vi "AcqLoop.vi"(8 "error in (no error)":errorcluster, 11 "Device in":refnum<class "Device.lvclass">) -> (0 "error out":errorcluster, 3 "Device out":refnum<class "Device.lvclass">)   [LabVIEW 2020, in "Device.lvlib" / "Device.lvclass"]
uses:
  Device.lvclass
  C:/Program Files/National Instruments/LabVIEW 2020/vi.lib/ActorFramework/Actor/Actor.lvclass
  DeviceStatus.ctl
  Device.lvclass/Device.ctl
  <vilib>/ActorFramework/Actor/Actor.lvclass/Actor.ctl
  <vilib>/ActorFramework/Message Enqueuer/Message Enqueuer.lvclass/Message Enqueuer.ctl
  <vilib>/ActorFramework/Message Enqueuer/Init from Existing Queue.vi
  <vilib>/ActorFramework/Message Enqueuer/Enqueue.vi
  Device Messages/AcqLoop Msg/AcqLoop Msg.lvclass
  C:/Program Files/National Instruments/LabVIEW 2020/vi.lib/ActorFramework/Message/Message.lvclass
  <vilib>/ActorFramework/Message Priority Queue/Priority Enqueue.vi
  <vilib>/ActorFramework/Message Enqueuer/Message Enqueuer.lvclass
  <vilib>/ActorFramework/Actor/Actor.lvclass
  Device.lvlib
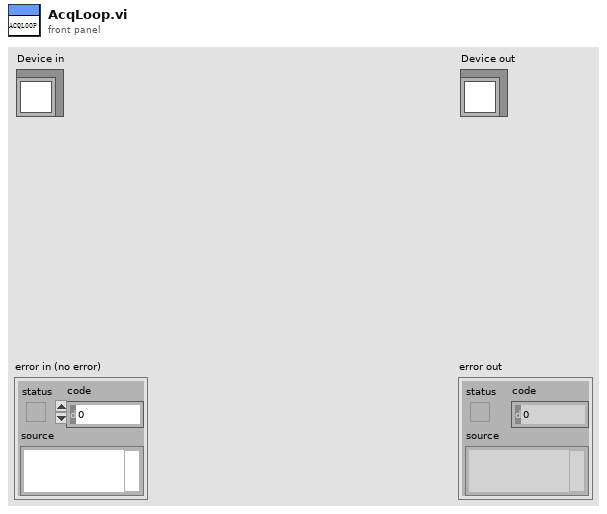
[diagram p1: front panel]
types:
  T1 = typedef "DataListener.lvclass/DataExchange.ctl" = cluster{"Source":string, "Destination":string, "Description":string, "value":variant}
  T2 = typedef "Device.lvlib/DeviceStatus.ctl" = i32
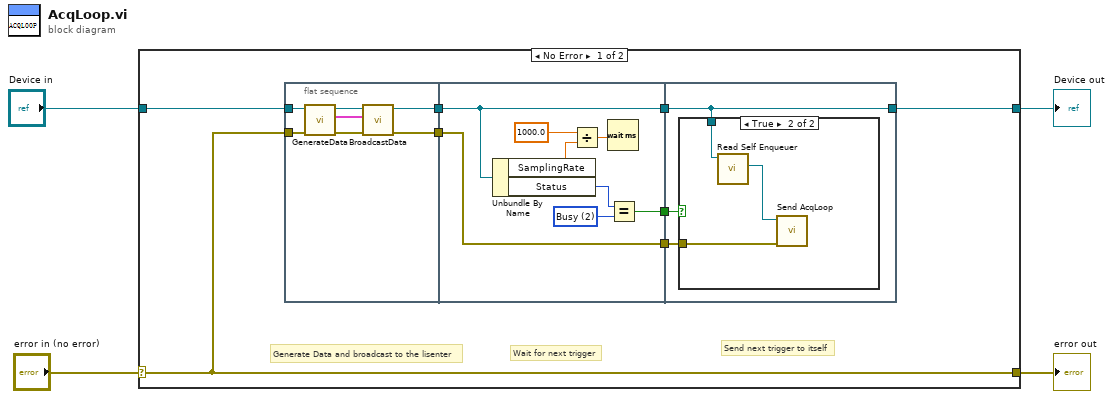
[diagram p0: block diagram]
diagram:
  n1 = case shown="No Error" "error in (no error)" {
    selector: "error in (no error)" -> [w7 w35]
    tunnel: [w7 w35] -> w3
    tunnel: [w5 w34] -> w1
    tunnel: "Device in" -> [w6 w34]
    frame No Error {
      # "Send next trigger to itself"
      # "Wait for next trigger"
      # "Generate Data and broadcast to the lisenter"
      n2 = flat-sequence {
        tunnel: w6 -> [w19]
        tunnel: w7 -> [w17]
        tunnel: [w16] -> w12
        tunnel: [w13] -> w11
        tunnel: w12 -> [w27]
        tunnel: [w27] -> w10
        tunnel: w11 -> [w21]
        tunnel: [w22] -> w9
        tunnel: [w21] -> w8
        tunnel: [w29] -> w5
        tunnel: w10 -> [w29]
        tunnel: w9 -> [w30]
        tunnel: w8 -> [w28]
        frame #0 {
          n3 = call-dynamic "GenerateData.vi"("error in (no error)"=w17, "Device in"=w19) -> ("error out"=w14:errorcluster, "DataExchange"=w15:T1, "Device out"=w18:refnum<class "Device.lvclass">)  [unwired: 7 in]
          n4 = call-dynamic "BroadcastData.vi"("error in (no error)"=w14, "DataExchange"=w15, "Device in"=w18) -> ("error out"=w13:errorcluster, "Device out"=w16:refnum<class "Device.lvclass">)  [unwired: 7 in]
        }
        frame #1 {
          w20 = T2 2 items=["Offline", "Idle", "Busy"] ("y")
          n5 = Unbundle By Name(w27) -> ("SamplingRate"=w26:dbl, "Status"=w23:T2)
          n6 = Divide(x=1000.0, y=w26) -> (x/y=w24:dbl)
          n7 = Wait (ms)(milliseconds to wait=w24) -> ()  [unwired: 1 out]
          n8 = Equal?(x=w23, y=w20) -> (x = y?=w22:bool)
        }
        frame #2 {
          n9 = case shown="True" w30 {
            tunnel: w29 -> [_ w33]
            tunnel: w28 -> [_ w31]
            frame False {
            }
            frame True {
              n10 = call <vilib>:"Read Self Enqueuer.vi"("Actor"=w33) -> ("Self Enqueuer"=w32:refnum<class "Message Enqueuer.lvclass">)  [unwired: 10 in]
              n11 = call "Send AcqLoop.vi"("error in (no error)"=w31, "Message Enqueuer"=w32) -> ()  [unwired: 8 in, 2 out]
            }
          }
        }
      }
    }
    frame Error {
    }
  }
  "error out" <- w3
  "Device out" <- w1
